vi "load methods.vi"(8 "error in (no error)":errorcluster, 11 "Folder Path":path) -> (0 "error out":errorcluster, 3 "Variant":variant)   [LabVIEW 2017]
uses:
  <vilib>/NI/JSON Support for LabVIEW/JSON Value/JSON Value.lvclass
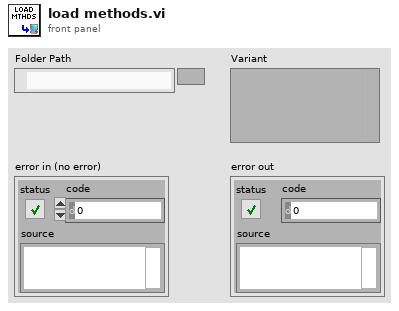
[diagram p1: front panel]
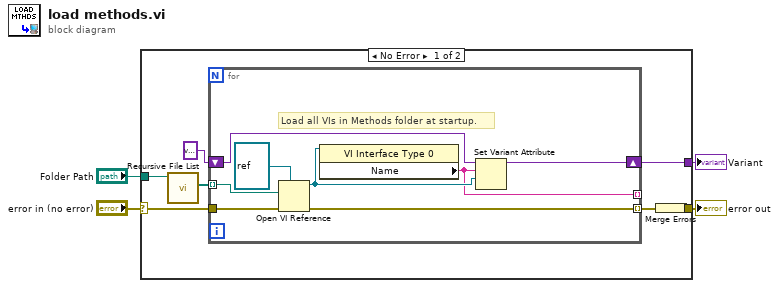
[diagram p0: block diagram]
diagram:
  n1 = case shown="No Error" "error in (no error)" {
    selector: "error in (no error)" -> [w5 w20]
    tunnel: [w11 _] -> w4
    tunnel: [w8 w20] -> w3
    tunnel: "Folder Path" -> [w7 _]
    frame No Error {
      n2 = call <vilib>:"Recursive File List.vi"("Folder Path"=w7) -> ("All Files in Dir"=w6:path[])  [unwired: 6 in, 4 out]
      n3 = for {
        tunnel: w6 -> [w19] mode=indexing
        tunnel: [w18] -> w9 mode=indexing
        shift-right: [w17] -> w11
        shift-left: variant -> [w16]
        tunnel: [w14] -> _ mode=indexing
        tunnel: w5 -> [w12]
        # "Load all VIs in Methods folder at startup."
        n4 = Open VI Reference(type specifier VI Refnum (for type only)=refnum<vi> refnum, vi path=w19, error in (no error)=w12) -> (vi reference=w15:refnum<vi>, error out=w18:errorcluster)  [unwired: 3 in]
        n5 = property class="VI Interface Type 0"(reference=w15) -> ("Name"=w14:string)  [unwired: 1 in, 2 out]
        n6 = Set Variant Attribute(Variant=w16, name=w14, value=w15) -> (Variant out=w17:variant)  [unwired: 1 in, 2 out]
      }
      n7 = Merge Errors(w9) -> (w8:errorcluster)
    }
    frame Error {
    }
  }
  "Variant" <- w4
  "error out" <- w3
